vi "Autonomous Independent.vi"() -> ()   [LabVIEW 2020]
doc: "This VI is called when autonomous begins, and will automatically be terminated when autonomous ends. You can carry out timed or sensor driven robot movement independently without needing to return to the caller."
uses:
  <vilib>/Rock Robotics/WPI/ThirdParty/Phoenix-LabVIEW/Motor Controller/Controls/CTRE_Phoenix_MotorControl_ControlMode.ctl
  <vilib>/Rock Robotics/WPI/Utilities/WPI_GetSetVariantRefNum.vi
  <vilib>/Rock Robotics/Network Tables/NT Read String.vi
  <vilib>/Rock Robotics/Network Tables/NT Write Numeric Array.vi
  <vilib>/Rock Robotics/WPI/ThirdParty/Phoenix-LabVIEW/Motor Controller/Get/CTRE_Phoenix_MotorController_GetSelectedSensorData.vi
  <vilib>/Rock Robotics/WPI/RobotDrive/WPI_RobotDriveArcadeDrive_Standard(NoSaturation).vi
panel:
  out "Talon FX LEFT Moter Encoders":i32
  out "Current Movement, for debugging":T1 {"Y Joystick Value" scale=1.0..-1.0; "X Joystick Value" scale=-1.0..1.0}
  in  "Array of robot movements":T2(array[cluster])=[{"X Joystick Value"=0.39393939393939403, "Y Joystick Value"=0.0, "Delay (sec)"=1.0, "Movement Name"="turn"}, {"X Joystick Value"=-0.3737373737373737, "Y Joystick Value"=0.0, "Delay (sec)"=1.0, "Movement Name"="turn back"}] {"Y Joystick Value" scale=1.0..-1.0; "X Joystick Value" scale=-1.0..1.0}
  # "Be sure to right-click and choose Data Operations>>Make Current Value default if you want to save the array values with the VI"
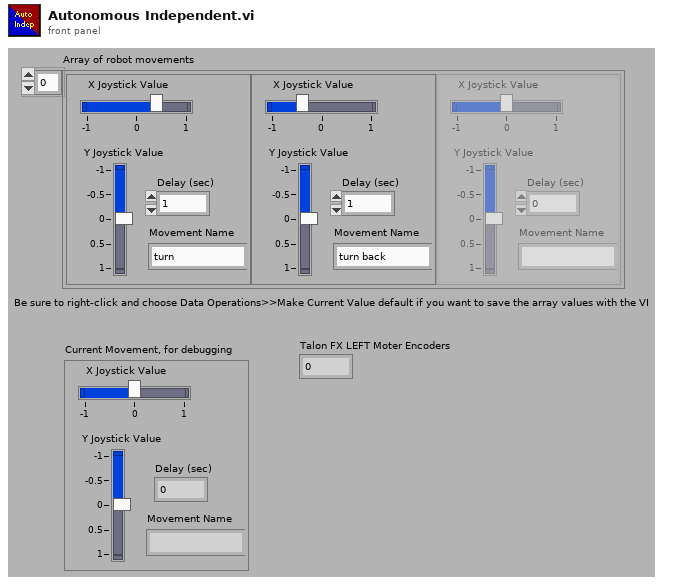
[diagram p1: front panel]
types:
  T1 = cluster{"X Joystick Value":dbl, "Y Joystick Value":dbl, "Delay (sec)":dbl, "Movement Name":string}
  T2 = cluster{"X Joystick Value":dbl, "Y Joystick Value":dbl, "Delay (sec)":dbl, "Movement Name":string}[]
  T3 = typedef "WPI_JoystickDevRef.ctl" = cluster{"Device":T4}
  T4 = typedef "WPI_JoystickDeviceEnum.ctl" = enum16{"USB 0", "USB 1", "USB 2", "USB 3", "USB 4", "USB 5"}
  T5 = typedef "WPI_MotorControlDeviceRef.ctl" = cluster{"DeviceStatus":errorcluster, "Type":T6, "PWM":cluster{"PWM Channel":T7, "DeadBand":T8}, "CAN":cluster{"Device Number":u8, "SetOutput VI Ref":variant, "GetOutput VI Ref":variant, "Enable VI Ref":variant, "Disable VI Ref":variant, "Data":variant}, "Invert":bool, "DIO PWM":cluster{"PWM \"Enable\" Channel":T7, "DIOChannel":T9, "PWM Rate":dbl}}
  T6 = typedef "WPI_MotorControlType.ctl" = enum16{"PWM", "CAN", "DIO PWM"}
  T7 = typedef "FPGA_DIOPWMChannel.ctl" = enum8{"PWM 0", "PWM 1", "PWM 2", "PWM 3", "PWM 4", "PWM 5", "PWM 6", "PWM 7", "PWM 8", "PWM 9", "PWM MXP 0", "PWM MXP 1", "PWM MXP 2", "PWM MXP 3", "PWM MXP 4", "PWM MXP 5", "PWM MXP 6", "PWM MXP 7", "PWM MXP 8", "PWM MXP 9", "Invalid"}
  T8 = typedef "WPI_PWMDeadband.ctl" = cluster{"Name":string, "maxPositivePwm":i32, "minPositivePwm":i32, "centerPwm":i32, "maxNegativePwm":i32, "minNegativePwm":i32, "angularRange":u16}
  T9 = typedef "FPGA_DIOChannel.ctl" = enum8{"DIO 0", "DIO 1", "DIO 2", "DIO 3", "DIO 4", "DIO 5", "DIO 6", "DIO 7", "DIO 8", "DIO 9", "DIO MXP 0", "DIO MXP 1", "DIO MXP 2", "DIO MXP 3", "DIO MXP 4", "DIO MXP 5", "DIO MXP 6", "DIO MXP 7", "DIO MXP 8", "DIO MXP 9", "DIO MXP 10", "DIO MXP 11", "DIO MXP 12", "DIO MXP 13", "DIO MXP 14", "DIO MXP 15", "SPI Port CS1", "SPI Port CS2", "SPI Port CS3", "SPI Port MISO", "SPI Port MOSI", "Invalid"}
  T10 = typedef "WPI_RobotDriveDevRef.ctl" = cluster{"DevStatus":errorcluster, "Motors[]":T5[], "Square Inputs":bool, "Max Output":dbl}
  T11 = typedef "CTRE_Phoenix_MotorControl_ControlMode.ctl" = u16
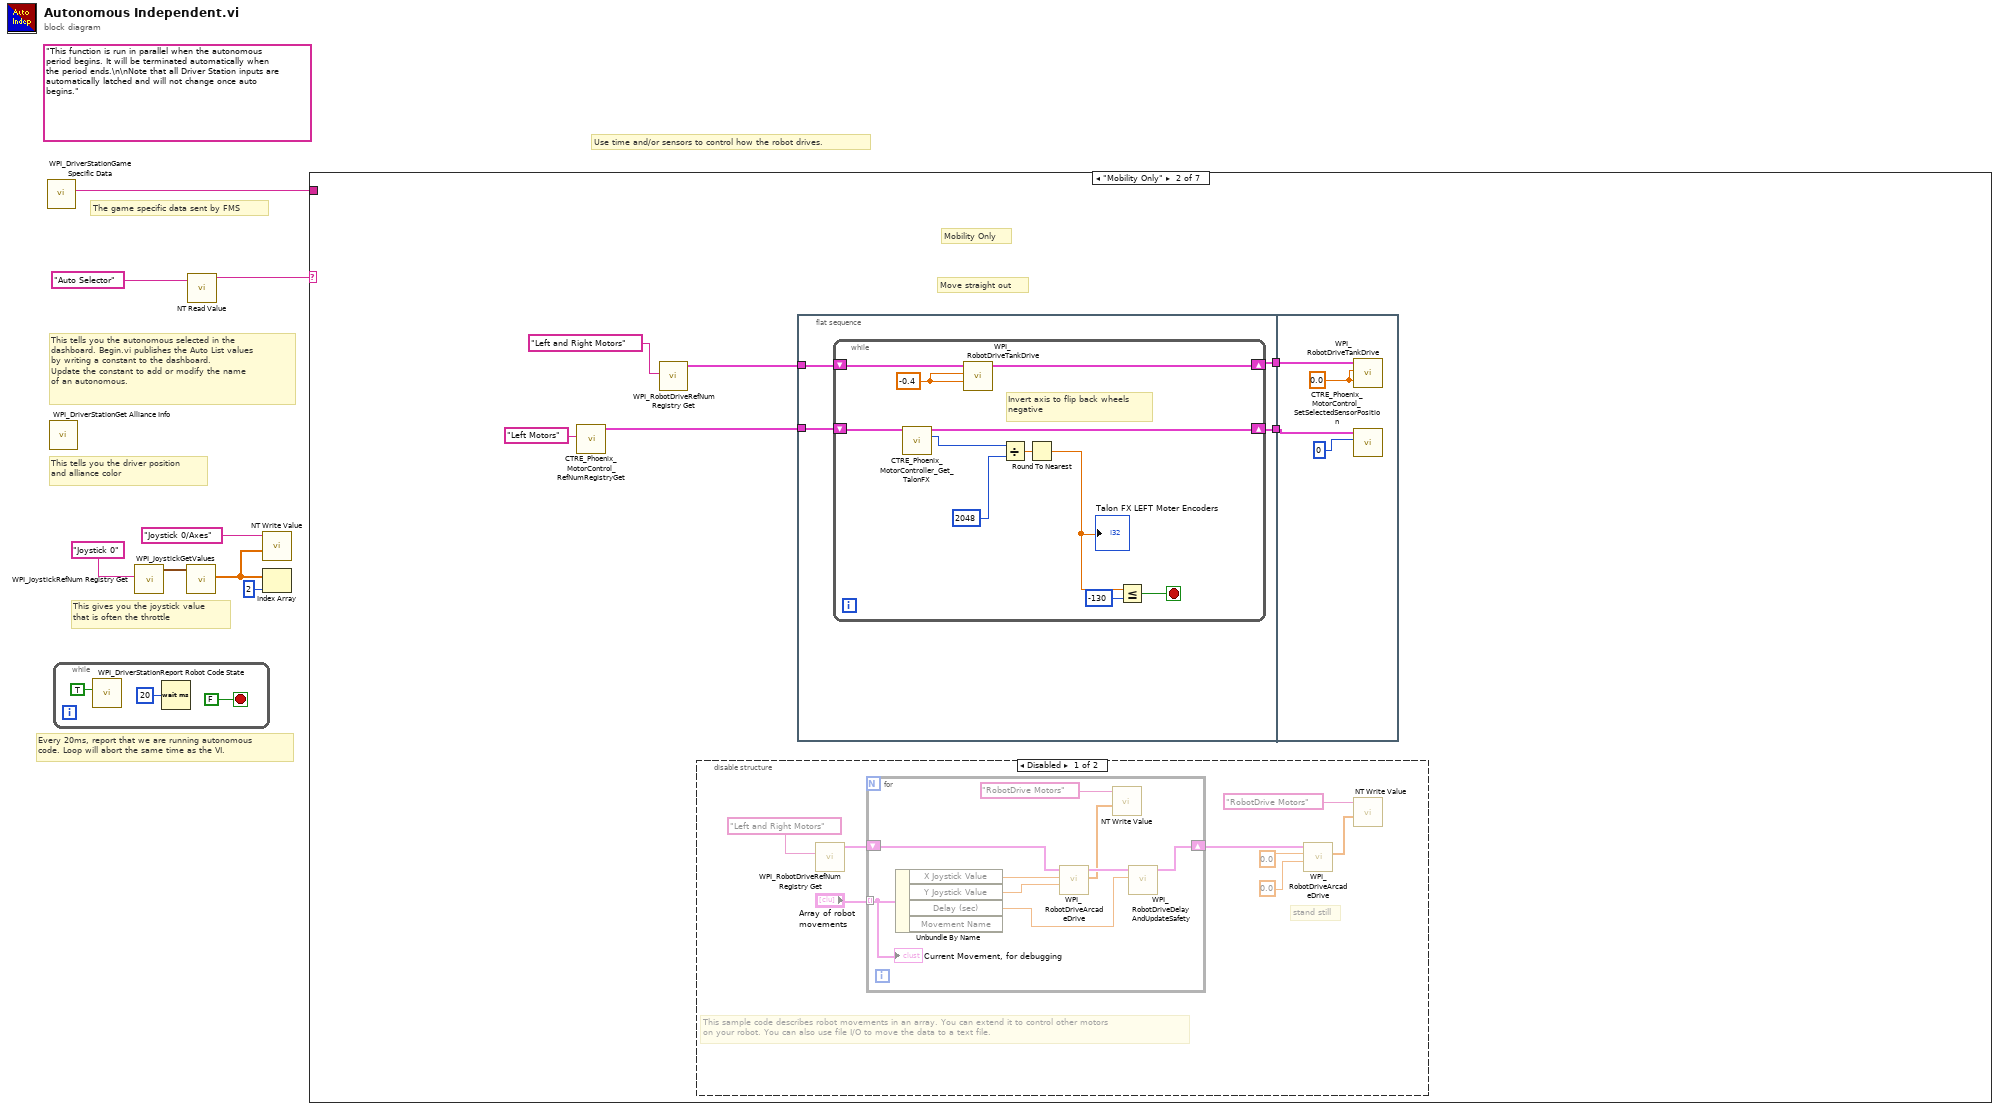
[diagram p0: block diagram]
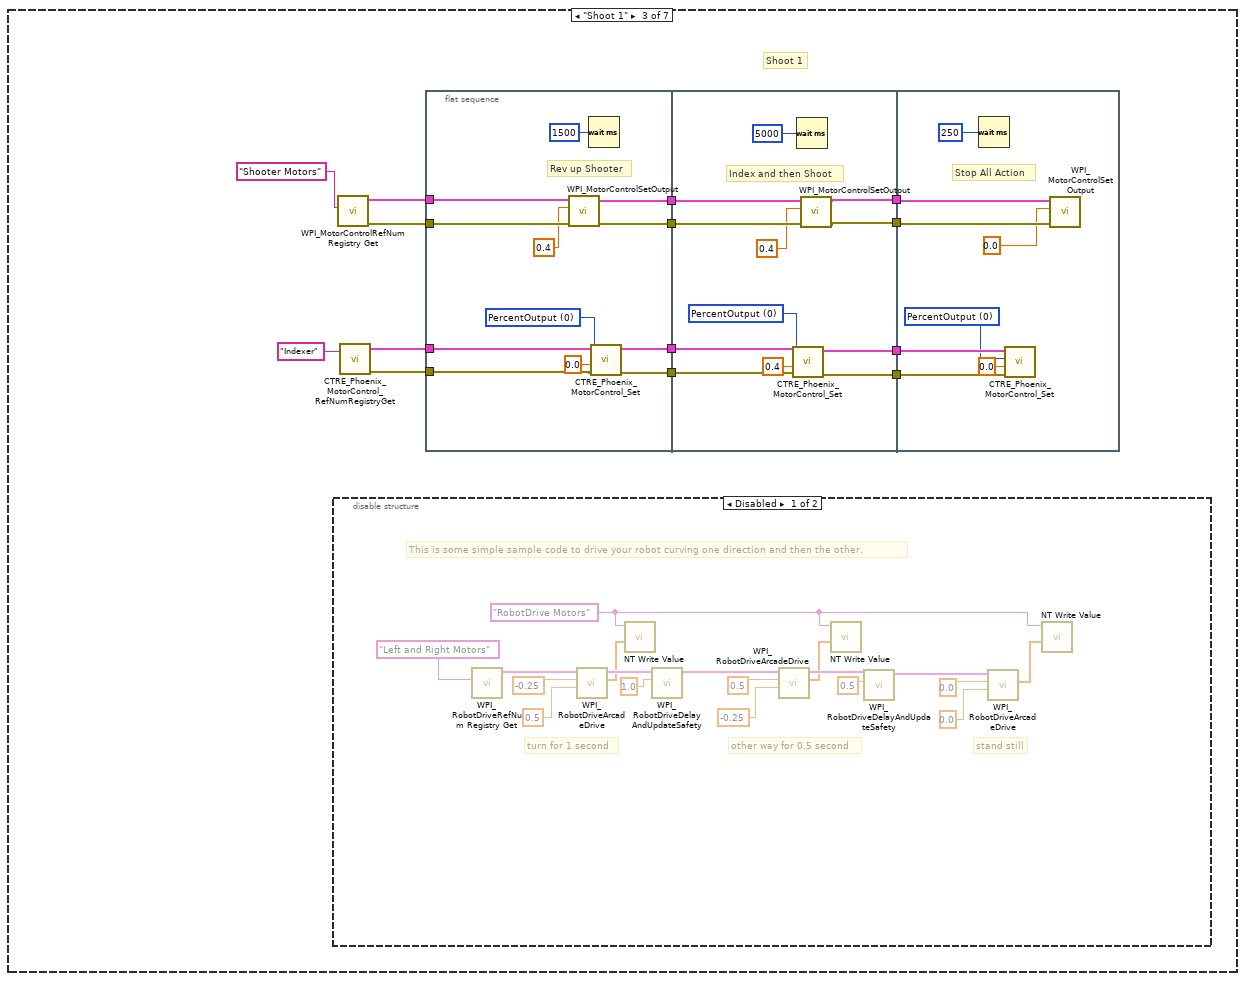
[diagram p4: hidden frame]
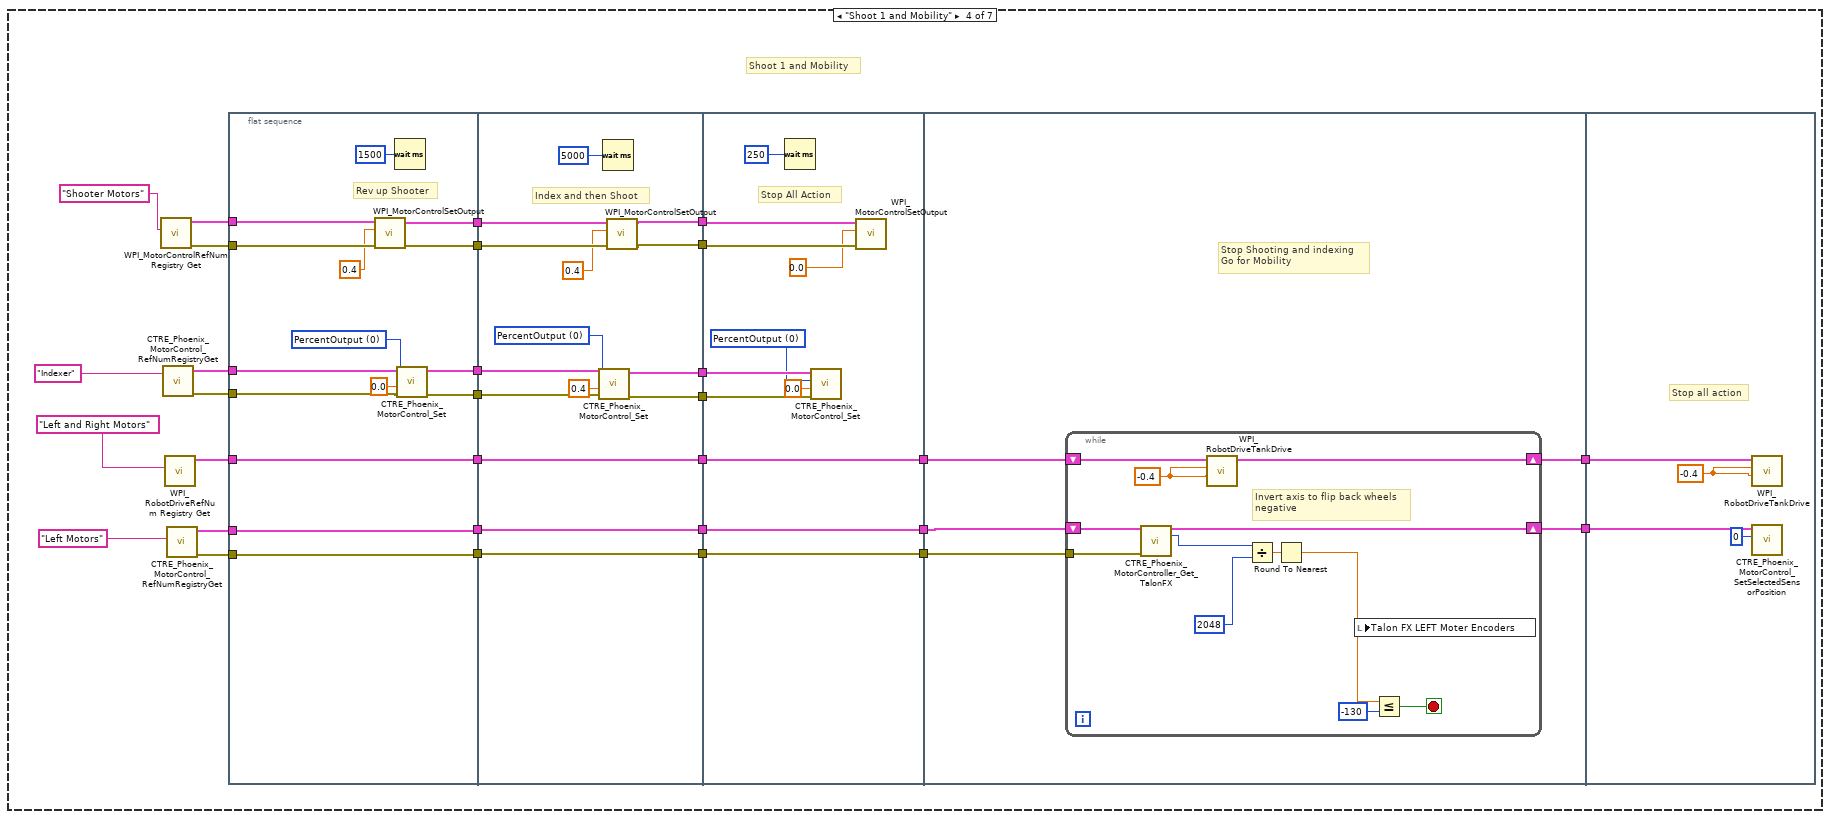
[diagram p6: hidden frame]
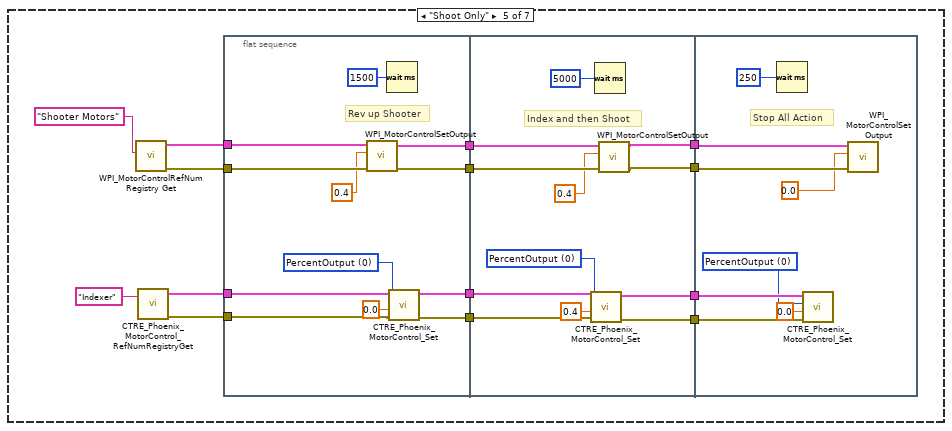
[diagram p7: hidden frame]
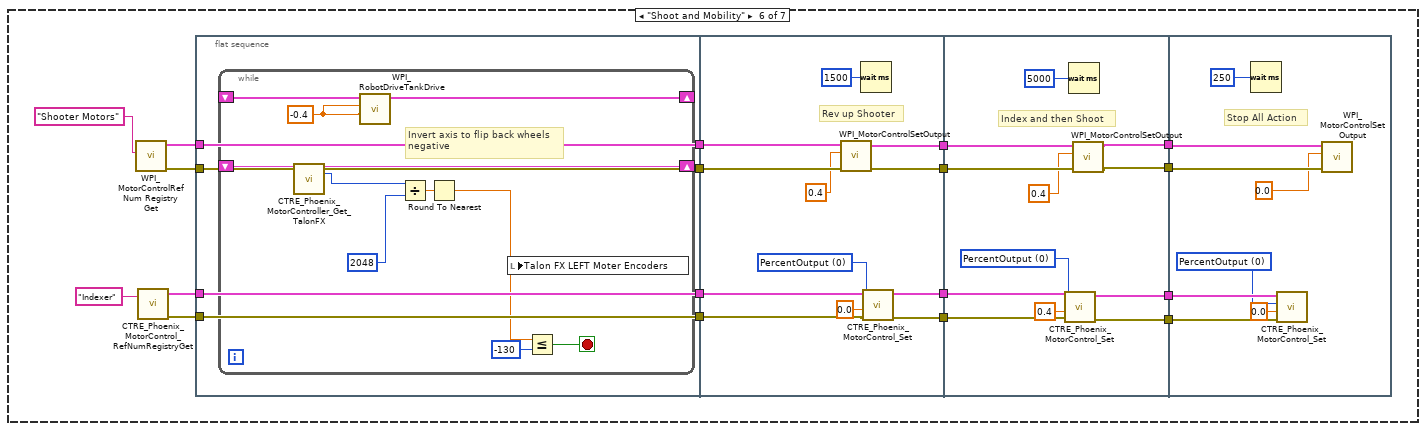
[diagram p8: hidden frame]
diagram:
  (unwired) "This function is run in parallel when the autonomous period begins. It will be terminated automatically when the period ends.\n\nNote that all Driver Station inputs are automatically latched and will not change once auto begins."
  # "The game specific data sent by FMS"
  # "This tells you the autonomous selected in the \ndashboard. Begin.vi publishes the Auto List values\nby writing a constant to the dashboard.\nUpdate the constant to add or modify the name\nof an autonomous."
  # "Every 20ms, report that we are running autonomous\ncode. Loop will abort the same time as the VI."
  # "This gives you the joystick value\nthat is often the throttle"
  # "Use time and/or sensors to control how the robot drives."
  # "This tells you the driver position\nand alliance color"
  n1 = call <vilib>:"WPI_DriverStationGame Specific Data.vi"() -> ("Game Specific Data"=w1:string)  [unwired: 11 in]
  n2 = call <vilib>:"WPI_DriverStationGet Alliance Info.vi"() -> ()  [unwired: 12 out]
  n3 = while {
    stop <- FALSE stop-if-true
    n4 = call <vilib>:"WPI_DriverStationReport Robot Code State.vi"("Autonomous"=TRUE) -> ()  [unwired: 10 in, 1 out]
    n5 = Wait (ms)(milliseconds to wait=u32 20) -> ()  [unwired: 1 out]
  }
  n6 = call <vilib>:"WPI_JoystickRefNum Registry Get.vi"("refnum name"="Joystick 0") -> ("JoystickDevRef"=w7:T3)  [unwired: 1 in, 9 out]
  n7 = call <vilib>:"WPI_JoystickGetValues.vi"("JoystickDevRef"=w7) -> ("Axes"=w3:dbl[])  [unwired: 6 in, 4 out]
  n8 = call-poly <vilib>:"NT Read Value.vi"("name"="Auto Selector" ("Name")) -> ("value"=w4:string)  [unwired: 8 in, 2 out]
  n9 = call-poly <vilib>:"NT Write Value.vi"("value"=w3, "name"="Joystick 0/Axes" ("Name")) -> ()  [unwired: 9 in, 1 out]
  n10 = Index Array(array=w3, index=2) -> ()  [unwired: 1 out]
  n11 = case shown="\"Mobility Only\"" w4 {
    tunnel: w1 -> [_ _ _ _ _ _ _]
    frame Default {
      # "You can put your main auto here, or you can right-click on the case and make any\nother frame be the default case."
      # "This is the frame that will execute if no selection is made, or if it is not recognized"
    }
    frame "Mobility Only" {
      # "Mobility Only"
      # "Move straight out"
      n12 = call <vilib>:"CTRE_Phoenix_MotorControl_RefNumRegistryGet.vi"("refnum name"="Left Motors") -> ("PhoenixMotorControlDevRef"=w14:T5)  [unwired: 9 in, 1 out]
      n13 = call <vilib>:"WPI_RobotDriveRefNum Registry Get.vi"("refnum name"="Left and Right Motors") -> ("RobotDriveDevRef"=w15:T10)  [unwired: 9 in, 1 out]
      n14 = disable-structure shown="Disabled" {
        frame Disabled {
          # "stand still"
          # "This sample code describes robot movements in an array. You can extend it to control other motors\non your robot. You can also use file I/O to move the data to a text file."
          n15 = call <vilib>:"WPI_RobotDriveRefNum Registry Get.vi"("refnum name"="Left and Right Motors") -> ("RobotDriveDevRef"=w43:T10)  [unwired: 1 in, 9 out]
          n16 = for {
            shift-right: [w51] -> w38
            shift-left: w43 -> [w52]
            tunnel: "Array of robot movements" -> [w47] mode=indexing
            n17 = Unbundle By Name(w47) -> ("X Joystick Value"=w50:dbl, "Y Joystick Value"=w49:dbl, "Delay (sec)"=w48:dbl)  [unwired: 1 out]
            n18 = call-poly <vilib>:"WPI_RobotDriveArcadeDrive.vi"("Y axis value"=w49, "X axis value"=w50, "RobotDriveDevRef"=w52) -> ("Motor Values"=w45:dbl[], "RobotDriveDevRef"=w53:T10)  [unwired: 1 in, 6 out]
            n19 = call-poly <vilib>:"NT Write Value.vi"("value"=w45, "name"="RobotDrive Motors" ("Name")) -> ()  [unwired: 9 in, 1 out]
            n20 = call <vilib>:"WPI_RobotDriveDelayAndUpdateSafety.vi"("Delay (s)"=w48, "RobotDriveDevRef"=w53) -> ("RobotDriveDevRef 2"=w51:T10)  [unwired: 8 in, 1 out]
            "Current Movement, for debugging" <- w47
          }
          n21 = call-poly <vilib>:"WPI_RobotDriveArcadeDrive.vi"("Y axis value"=0.0 ("X axis value"), "X axis value"=0.0, "RobotDriveDevRef"=w38) -> ("Motor Values"=w41:dbl[])  [unwired: 1 in, 7 out]
          n22 = call-poly <vilib>:"NT Write Value.vi"("value"=w41, "name"="RobotDrive Motors" ("Name")) -> ()  [unwired: 9 in, 1 out]
        }
        frame Enabled {
        }
      }
      n23 = flat-sequence {
        tunnel: w15 -> [w21]
        tunnel: [w20] -> w17
        tunnel: [w19] -> w16
        tunnel: w14 -> [w18]
        tunnel: w17 -> [w35]
        tunnel: w16 -> [w34]
        frame #0 {
          n24 = while {
            shift-right: [w30] -> w20
            shift-left: w21 -> [w32]
            shift-right: [w29] -> w19
            shift-left: w18 -> [w31]
            stop <- w28 stop-if-true
            w27 = -0.4 ("Left axis value")
            # "Invert axis to flip back wheels\nnegative"
            n25 = call-poly <vilib>:"CTRE_Phoenix_MotorController_Get_TalonFX.vi"("PhoenixMotorControlDevRef"=w31) -> ("PhoenixMotorControlDevRef"=w29:T5, "Position (Raw Sensor Units)"=w23:i32)  [unwired: 11 in, 2 out]
            n26 = call <vilib>:"WPI_RobotDriveTankDrive.vi"("Right axis value"=w27, "Left axis value"=w27, "RobotDriveDevRef"=w32) -> ("RobotDriveDevRef"=w30:T10)  [unwired: 6 in, 2 out]
            n27 = Divide(x=w23, y=2048) -> (x/y=w24:dbl)
            n28 = Round To Nearest(number=w24) -> (nearest integer value=w22:dbl)
            "Talon FX LEFT Moter Encoders" <- w22
            n29 = Less Or Equal?(x=w22, y=-130) -> (x <= y?=w28:bool)
          }
        }
        frame #1 {
          w36 = 0.0
          n30 = call <vilib>:"WPI_RobotDriveTankDrive.vi"("Right axis value"=w36, "Left axis value"=w36, "RobotDriveDevRef"=w35) -> ()  [unwired: 6 in, 3 out]
          n31 = call <vilib>:"CTRE_Phoenix_MotorControl_SetSelectedSensorPosition.vi"("New Sensor Position"=0, "PhoenixMotorControlDevRef"=w34) -> ()  [unwired: 8 in, 2 out]
        }
      }
    }
    frame "Shoot 1" {
      # "Shoot 1"
      n32 = disable-structure shown="Disabled" {
        frame Disabled {
          w101 = "RobotDrive Motors" ("Name")
          # "This is some simple sample code to drive your robot curving one direction and then the other."
          # "stand still"
          # "other way for 0.5 second"
          # "turn for 1 second"
          n33 = call <vilib>:"WPI_RobotDriveRefNum Registry Get.vi"("refnum name"="Left and Right Motors") -> ("RobotDriveDevRef"=w117:T10)  [unwired: 1 in, 9 out]
          n34 = call-poly <vilib>:"WPI_RobotDriveArcadeDrive.vi"("Y axis value"=0.5 ("X axis value"), "X axis value"=-0.25, "RobotDriveDevRef"=w117) -> ("Motor Values"=w100:dbl[], "RobotDriveDevRef"=w110:T10)  [unwired: 1 in, 6 out]
          n35 = call-poly <vilib>:"NT Write Value.vi"("value"=w100, "name"=w101) -> ()  [unwired: 9 in, 1 out]
          n36 = call <vilib>:"WPI_RobotDriveDelayAndUpdateSafety.vi"("Delay (s)"=1.0, "RobotDriveDevRef"=w110) -> ("RobotDriveDevRef 2"=w111:T10)  [unwired: 8 in, 1 out]
          n37 = call-poly <vilib>:"WPI_RobotDriveArcadeDrive.vi"("Y axis value"=-0.25 ("X axis value"), "X axis value"=0.5, "RobotDriveDevRef"=w111) -> ("Motor Values"=w102:dbl[], "RobotDriveDevRef"=w112:T10)  [unwired: 1 in, 6 out]
          n38 = call-poly <vilib>:"NT Write Value.vi"("value"=w102, "name"=w101) -> ()  [unwired: 9 in, 1 out]
          n39 = call <vilib>:"WPI_RobotDriveDelayAndUpdateSafety.vi"("Delay (s)"=0.5, "RobotDriveDevRef"=w112) -> ("RobotDriveDevRef 2"=w113:T10)  [unwired: 8 in, 1 out]
          n40 = call-poly <vilib>:"WPI_RobotDriveArcadeDrive.vi"("Y axis value"=0.0 ("X axis value"), "X axis value"=0.0, "RobotDriveDevRef"=w113) -> ("Motor Values"=w103:dbl[])  [unwired: 1 in, 7 out]
          n41 = call-poly <vilib>:"NT Write Value.vi"("value"=w103, "name"=w101) -> ()  [unwired: 9 in, 1 out]
        }
        frame Enabled {
        }
      }
      n42 = call <vilib>:"WPI_MotorControlRefNum Registry Get.vi"("refnum name"="Shooter Motors") -> ("error out"=w56:errorcluster, "MotorControlDevRef"=w57:T5)  [unwired: 9 in]
      n43 = call <vilib>:"CTRE_Phoenix_MotorControl_RefNumRegistryGet.vi"("refnum name"="Indexer") -> ("error out"=w58:errorcluster, "PhoenixMotorControlDevRef"=w59:T5)  [unwired: 9 in]
      n44 = flat-sequence {
        tunnel: w57 -> [w79]
        tunnel: w56 -> [w78]
        tunnel: [w75] -> w67
        tunnel: [w74] -> w66
        tunnel: [w73] -> w65
        tunnel: [w72] -> w64
        tunnel: w59 -> [w71]
        tunnel: w58 -> [w70]
        tunnel: w67 -> [w90]
        tunnel: w66 -> [w89]
        tunnel: [w88] -> w63
        tunnel: [w87] -> w62
        tunnel: [w85] -> w61
        tunnel: [w84] -> w60
        tunnel: w65 -> [w83]
        tunnel: w64 -> [w82]
        tunnel: w63 -> [w99]
        tunnel: w62 -> [w98]
        tunnel: w61 -> [w95]
        tunnel: w60 -> [w94]
        frame #0 {
          w68 = T11 0 items=["PercentOutput"=0, "Position"=1, "Velocity"=2, "Current"=3, "Follower"=5, "MotionProfile"=6, "MotionMagic"=7, "MotionProfileArc"=10, "Disabled"=15] ("Control Mode")
          # "Rev up Shooter"
          n45 = call <vilib>:"WPI_MotorControlSetOutput.vi"("error in (no error)"=w78, "Output"=0.4, "MotorControlDevRef"=w79) -> ("error out"=w74:errorcluster, "MotorControlDevRef"=w75:T5)  [unwired: 6 in, 1 out]
          n46 = Wait (ms)(milliseconds to wait=u32 1500) -> ()  [unwired: 1 out]
          n47 = call <vilib>:"CTRE_Phoenix_MotorControl_Set.vi"("error in (no error)"=w70, "Output"=0.0, "Control Mode"=w68, "PhoenixMotorControlDevRef"=w71) -> ("error out"=w72:errorcluster, "PhoenixMotorControlDevRef"=w73:T5)  [unwired: 6 in]
        }
        frame #1 {
          w80 = T11 0 items=["PercentOutput"=0, "Position"=1, "Velocity"=2, "Current"=3, "Follower"=5, "MotionProfile"=6, "MotionMagic"=7, "MotionProfileArc"=10, "Disabled"=15] ("Control Mode")
          # "Index and then Shoot"
          n48 = call <vilib>:"CTRE_Phoenix_MotorControl_Set.vi"("error in (no error)"=w82, "Output"=0.4, "Control Mode"=w80, "PhoenixMotorControlDevRef"=w83) -> ("error out"=w84:errorcluster, "PhoenixMotorControlDevRef"=w85:T5)  [unwired: 6 in]
          n49 = Wait (ms)(milliseconds to wait=u32 5000) -> ()  [unwired: 1 out]
          n50 = call <vilib>:"WPI_MotorControlSetOutput.vi"("error in (no error)"=w89, "Output"=0.4, "MotorControlDevRef"=w90) -> ("error out"=w87:errorcluster, "MotorControlDevRef"=w88:T5)  [unwired: 6 in, 1 out]
        }
        frame #2 {
          w92 = T11 0 items=["PercentOutput"=0, "Position"=1, "Velocity"=2, "Current"=3, "Follower"=5, "MotionProfile"=6, "MotionMagic"=7, "MotionProfileArc"=10, "Disabled"=15] ("Control Mode")
          # "Stop All Action"
          n51 = Wait (ms)(milliseconds to wait=u32 250) -> ()  [unwired: 1 out]
          n52 = call <vilib>:"CTRE_Phoenix_MotorControl_Set.vi"("error in (no error)"=w94, "Output"=0.0, "Control Mode"=w92, "PhoenixMotorControlDevRef"=w95) -> ()  [unwired: 6 in, 2 out]
          n53 = call <vilib>:"WPI_MotorControlSetOutput.vi"("error in (no error)"=w98, "Output"=0.0, "MotorControlDevRef"=w99) -> ()  [unwired: 6 in, 3 out]
        }
      }
    }
    frame "Shoot 1 and Mobility" {
      # "Shoot 1 and Mobility"
      n54 = call <vilib>:"WPI_MotorControlRefNum Registry Get.vi"("refnum name"="Shooter Motors") -> ("error out"=w136:errorcluster, "MotorControlDevRef"=w137:T5)  [unwired: 9 in]
      n55 = call <vilib>:"CTRE_Phoenix_MotorControl_RefNumRegistryGet.vi"("refnum name"="Indexer") -> ("error out"=w138:errorcluster, "PhoenixMotorControlDevRef"=w139:T5)  [unwired: 9 in]
      n56 = call <vilib>:"WPI_RobotDriveRefNum Registry Get.vi"("refnum name"="Left and Right Motors") -> ("RobotDriveDevRef"=w130:T10)  [unwired: 9 in, 1 out]
      n57 = call <vilib>:"CTRE_Phoenix_MotorControl_RefNumRegistryGet.vi"("refnum name"="Left Motors") -> ("error out"=w122:errorcluster, "PhoenixMotorControlDevRef"=w126:T5)  [unwired: 9 in]
      n58 = flat-sequence {
        tunnel: [w158] -> w147
        tunnel: [w157] -> w146
        tunnel: [w156] -> w145
        tunnel: [w155] -> w144
        tunnel: w137 -> [w162]
        tunnel: w136 -> [w161]
        tunnel: w139 -> [w154]
        tunnel: w138 -> [w153]
        tunnel: [w150] -> w131
        tunnel: w130 -> [w150]
        tunnel: [w149] -> w127
        tunnel: w126 -> [w149]
        tunnel: [w148] -> w123
        tunnel: w122 -> [w148]
        tunnel: w147 -> [w176]
        tunnel: w146 -> [w175]
        tunnel: [w174] -> w143
        tunnel: [w173] -> w142
        tunnel: [w171] -> w141
        tunnel: [w170] -> w140
        tunnel: w145 -> [w169]
        tunnel: w144 -> [w168]
        tunnel: w131 -> [w165]
        tunnel: [w165] -> w129
        tunnel: w127 -> [w164]
        tunnel: [w164] -> w125
        tunnel: w123 -> [w163]
        tunnel: [w163] -> w120
        tunnel: w143 -> [w188]
        tunnel: w142 -> [w187]
        tunnel: w141 -> [w184]
        tunnel: w140 -> [w183]
        tunnel: w129 -> [w180]
        tunnel: [w180] -> w128
        tunnel: w125 -> [w179]
        tunnel: [w179] -> w124
        tunnel: [w178] -> w121
        tunnel: w120 -> [w178]
        tunnel: w128 -> [w193]
        tunnel: w124 -> [w192]
        tunnel: w121 -> [w191]
        tunnel: [w190] -> w119
        tunnel: [w189] -> w118
        tunnel: w119 -> [w208]
        tunnel: w118 -> [w207]
        frame #0 {
          w151 = T11 0 items=["PercentOutput"=0, "Position"=1, "Velocity"=2, "Current"=3, "Follower"=5, "MotionProfile"=6, "MotionMagic"=7, "MotionProfileArc"=10, "Disabled"=15] ("Control Mode")
          # "Rev up Shooter"
          n59 = call <vilib>:"WPI_MotorControlSetOutput.vi"("error in (no error)"=w161, "Output"=0.4, "MotorControlDevRef"=w162) -> ("error out"=w157:errorcluster, "MotorControlDevRef"=w158:T5)  [unwired: 6 in, 1 out]
          n60 = Wait (ms)(milliseconds to wait=u32 1500) -> ()  [unwired: 1 out]
          n61 = call <vilib>:"CTRE_Phoenix_MotorControl_Set.vi"("error in (no error)"=w153, "Output"=0.0, "Control Mode"=w151, "PhoenixMotorControlDevRef"=w154) -> ("error out"=w155:errorcluster, "PhoenixMotorControlDevRef"=w156:T5)  [unwired: 6 in]
        }
        frame #1 {
          w166 = T11 0 items=["PercentOutput"=0, "Position"=1, "Velocity"=2, "Current"=3, "Follower"=5, "MotionProfile"=6, "MotionMagic"=7, "MotionProfileArc"=10, "Disabled"=15] ("Control Mode")
          # "Index and then Shoot"
          n62 = call <vilib>:"CTRE_Phoenix_MotorControl_Set.vi"("error in (no error)"=w168, "Output"=0.4, "Control Mode"=w166, "PhoenixMotorControlDevRef"=w169) -> ("error out"=w170:errorcluster, "PhoenixMotorControlDevRef"=w171:T5)  [unwired: 6 in]
          n63 = Wait (ms)(milliseconds to wait=u32 5000) -> ()  [unwired: 1 out]
          n64 = call <vilib>:"WPI_MotorControlSetOutput.vi"("error in (no error)"=w175, "Output"=0.4, "MotorControlDevRef"=w176) -> ("error out"=w173:errorcluster, "MotorControlDevRef"=w174:T5)  [unwired: 6 in, 1 out]
        }
        frame #2 {
          w181 = T11 0 items=["PercentOutput"=0, "Position"=1, "Velocity"=2, "Current"=3, "Follower"=5, "MotionProfile"=6, "MotionMagic"=7, "MotionProfileArc"=10, "Disabled"=15] ("Control Mode")
          # "Stop All Action"
          n65 = Wait (ms)(milliseconds to wait=u32 250) -> ()  [unwired: 1 out]
          n66 = call <vilib>:"CTRE_Phoenix_MotorControl_Set.vi"("error in (no error)"=w183, "Output"=0.0, "Control Mode"=w181, "PhoenixMotorControlDevRef"=w184) -> ()  [unwired: 6 in, 2 out]
          n67 = call <vilib>:"WPI_MotorControlSetOutput.vi"("error in (no error)"=w187, "Output"=0.0, "MotorControlDevRef"=w188) -> ()  [unwired: 6 in, 3 out]
        }
        frame #3 {
          # "Stop Shooting and indexing\nGo for Mobility"
          n68 = while {
            shift-right: [w203] -> w190
            shift-left: w193 -> [w205]
            shift-right: [w202] -> w189
            shift-left: w192 -> [w204]
            tunnel: w191 -> [w194]
            stop <- w201 stop-if-true
            w200 = -0.4 ("Left axis value")
            # "Invert axis to flip back wheels\nnegative"
            n69 = call-poly <vilib>:"CTRE_Phoenix_MotorController_Get_TalonFX.vi"("PhoenixMotorControlDevRef"=w204, "error in"=w194) -> ("PhoenixMotorControlDevRef"=w202:T5, "Position (Raw Sensor Units)"=w196:i32)  [unwired: 10 in, 2 out]
            n70 = call <vilib>:"WPI_RobotDriveTankDrive.vi"("Right axis value"=w200, "Left axis value"=w200, "RobotDriveDevRef"=w205) -> ("RobotDriveDevRef"=w203:T10)  [unwired: 6 in, 2 out]
            n71 = Divide(x=w196, y=2048) -> (x/y=w197:dbl)
            n72 = Round To Nearest(number=w197) -> (nearest integer value=w195:dbl)
            n73 = local write "Talon FX LEFT Moter Encoders"(w195) -> ()
            n74 = Less Or Equal?(x=w195, y=-130) -> (x <= y?=w201:bool)
          }
        }
        frame #4 {
          w209 = -0.4 ("Left axis value")
          # "Stop all action"
          n75 = call <vilib>:"WPI_RobotDriveTankDrive.vi"("Right axis value"=w209, "Left axis value"=w209, "RobotDriveDevRef"=w208) -> ()  [unwired: 6 in, 3 out]
          n76 = call <vilib>:"CTRE_Phoenix_MotorControl_SetSelectedSensorPosition.vi"("New Sensor Position"=0, "PhoenixMotorControlDevRef"=w207) -> ()  [unwired: 8 in, 2 out]
        }
      }
    }
    frame "Shoot Only" {
      n77 = call <vilib>:"WPI_MotorControlRefNum Registry Get.vi"("refnum name"="Shooter Motors") -> ("error out"=w212:errorcluster, "MotorControlDevRef"=w213:T5)  [unwired: 9 in]
      n78 = call <vilib>:"CTRE_Phoenix_MotorControl_RefNumRegistryGet.vi"("refnum name"="Indexer") -> ("error out"=w214:errorcluster, "PhoenixMotorControlDevRef"=w215:T5)  [unwired: 9 in]
      n79 = flat-sequence {
        tunnel: w213 -> [w235]
        tunnel: w212 -> [w234]
        tunnel: [w231] -> w223
        tunnel: [w230] -> w222
        tunnel: [w229] -> w217
        tunnel: [w228] -> w216
        tunnel: w215 -> [w227]
        tunnel: w214 -> [w226]
        tunnel: w223 -> [w246]
        tunnel: w222 -> [w245]
        tunnel: [w244] -> w221
        tunnel: [w243] -> w220
        tunnel: [w241] -> w219
        tunnel: [w240] -> w218
        tunnel: w217 -> [w239]
        tunnel: w216 -> [w238]
        tunnel: w221 -> [w255]
        tunnel: w220 -> [w254]
        tunnel: w219 -> [w251]
        tunnel: w218 -> [w250]
        frame #0 {
          w224 = T11 0 items=["PercentOutput"=0, "Position"=1, "Velocity"=2, "Current"=3, "Follower"=5, "MotionProfile"=6, "MotionMagic"=7, "MotionProfileArc"=10, "Disabled"=15] ("Control Mode")
          # "Rev up Shooter"
          n80 = call <vilib>:"WPI_MotorControlSetOutput.vi"("error in (no error)"=w234, "Output"=0.4, "MotorControlDevRef"=w235) -> ("error out"=w230:errorcluster, "MotorControlDevRef"=w231:T5)  [unwired: 6 in, 1 out]
          n81 = Wait (ms)(milliseconds to wait=u32 1500) -> ()  [unwired: 1 out]
          n82 = call <vilib>:"CTRE_Phoenix_MotorControl_Set.vi"("error in (no error)"=w226, "Output"=0.0, "Control Mode"=w224, "PhoenixMotorControlDevRef"=w227) -> ("error out"=w228:errorcluster, "PhoenixMotorControlDevRef"=w229:T5)  [unwired: 6 in]
        }
        frame #1 {
          w236 = T11 0 items=["PercentOutput"=0, "Position"=1, "Velocity"=2, "Current"=3, "Follower"=5, "MotionProfile"=6, "MotionMagic"=7, "MotionProfileArc"=10, "Disabled"=15] ("Control Mode")
          # "Index and then Shoot"
          n83 = call <vilib>:"CTRE_Phoenix_MotorControl_Set.vi"("error in (no error)"=w238, "Output"=0.4, "Control Mode"=w236, "PhoenixMotorControlDevRef"=w239) -> ("error out"=w240:errorcluster, "PhoenixMotorControlDevRef"=w241:T5)  [unwired: 6 in]
          n84 = Wait (ms)(milliseconds to wait=u32 5000) -> ()  [unwired: 1 out]
          n85 = call <vilib>:"WPI_MotorControlSetOutput.vi"("error in (no error)"=w245, "Output"=0.4, "MotorControlDevRef"=w246) -> ("error out"=w243:errorcluster, "MotorControlDevRef"=w244:T5)  [unwired: 6 in, 1 out]
        }
        frame #2 {
          w248 = T11 0 items=["PercentOutput"=0, "Position"=1, "Velocity"=2, "Current"=3, "Follower"=5, "MotionProfile"=6, "MotionMagic"=7, "MotionProfileArc"=10, "Disabled"=15] ("Control Mode")
          # "Stop All Action"
          n86 = Wait (ms)(milliseconds to wait=u32 250) -> ()  [unwired: 1 out]
          n87 = call <vilib>:"CTRE_Phoenix_MotorControl_Set.vi"("error in (no error)"=w250, "Output"=0.0, "Control Mode"=w248, "PhoenixMotorControlDevRef"=w251) -> ()  [unwired: 6 in, 2 out]
          n88 = call <vilib>:"WPI_MotorControlSetOutput.vi"("error in (no error)"=w254, "Output"=0.0, "MotorControlDevRef"=w255) -> ()  [unwired: 6 in, 3 out]
        }
      }
    }
    frame "Shoot and Mobility" {
      n89 = call <vilib>:"WPI_MotorControlRefNum Registry Get.vi"("refnum name"="Shooter Motors") -> ("error out"=w262:errorcluster, "MotorControlDevRef"=w263:T5)  [unwired: 9 in]
      n90 = call <vilib>:"CTRE_Phoenix_MotorControl_RefNumRegistryGet.vi"("refnum name"="Indexer") -> ("error out"=w264:errorcluster, "PhoenixMotorControlDevRef"=w265:T5)  [unwired: 9 in]
      n91 = flat-sequence {
        tunnel: w264 -> [w274]
        tunnel: w265 -> [w275]
        tunnel: w262 -> [w276]
        tunnel: w263 -> [w277]
        tunnel: [w277] -> w259
        tunnel: [w276] -> w258
        tunnel: [w275] -> w257
        tunnel: [w274] -> w256
        tunnel: [w296] -> w273
        tunnel: [w295] -> w272
        tunnel: [w294] -> w271
        tunnel: [w293] -> w270
        tunnel: w259 -> [w300]
        tunnel: w258 -> [w299]
        tunnel: w257 -> [w292]
        tunnel: w256 -> [w291]
        tunnel: w273 -> [w311]
        tunnel: w272 -> [w310]
        tunnel: [w309] -> w269
        tunnel: [w308] -> w268
        tunnel: [w306] -> w267
        tunnel: [w305] -> w266
        tunnel: w271 -> [w304]
        tunnel: w270 -> [w303]
        tunnel: w269 -> [w320]
        tunnel: w268 -> [w319]
        tunnel: w267 -> [w316]
        tunnel: w266 -> [w315]
        frame #0 {
          n92 = while {
            shift-right: [w286] -> _
            shift-left: _ -> [w288]
            shift-right: [w285] -> _
            shift-left: _ -> [w287]
            stop <- w284 stop-if-true
            w283 = -0.4 ("Left axis value")
            # "Invert axis to flip back wheels\nnegative"
            n93 = call-poly <vilib>:"CTRE_Phoenix_MotorController_Get_TalonFX.vi"("PhoenixMotorControlDevRef"=w287) -> ("PhoenixMotorControlDevRef"=w285:T5, "Position (Raw Sensor Units)"=w279:i32)  [unwired: 11 in, 2 out]
            n94 = call <vilib>:"WPI_RobotDriveTankDrive.vi"("Right axis value"=w283, "Left axis value"=w283, "RobotDriveDevRef"=w288) -> ("RobotDriveDevRef"=w286:T10)  [unwired: 6 in, 2 out]
            n95 = Divide(x=w279, y=2048) -> (x/y=w280:dbl)
            n96 = Round To Nearest(number=w280) -> (nearest integer value=w278:dbl)
            n97 = local write "Talon FX LEFT Moter Encoders"(w278) -> ()
            n98 = Less Or Equal?(x=w278, y=-130) -> (x <= y?=w284:bool)
          }
        }
        frame #1 {
          w289 = T11 0 items=["PercentOutput"=0, "Position"=1, "Velocity"=2, "Current"=3, "Follower"=5, "MotionProfile"=6, "MotionMagic"=7, "MotionProfileArc"=10, "Disabled"=15] ("Control Mode")
          # "Rev up Shooter"
          n99 = call <vilib>:"WPI_MotorControlSetOutput.vi"("error in (no error)"=w299, "Output"=0.4, "MotorControlDevRef"=w300) -> ("error out"=w295:errorcluster, "MotorControlDevRef"=w296:T5)  [unwired: 6 in, 1 out]
          n100 = Wait (ms)(milliseconds to wait=u32 1500) -> ()  [unwired: 1 out]
          n101 = call <vilib>:"CTRE_Phoenix_MotorControl_Set.vi"("error in (no error)"=w291, "Output"=0.0, "Control Mode"=w289, "PhoenixMotorControlDevRef"=w292) -> ("error out"=w293:errorcluster, "PhoenixMotorControlDevRef"=w294:T5)  [unwired: 6 in]
        }
        frame #2 {
          w301 = T11 0 items=["PercentOutput"=0, "Position"=1, "Velocity"=2, "Current"=3, "Follower"=5, "MotionProfile"=6, "MotionMagic"=7, "MotionProfileArc"=10, "Disabled"=15] ("Control Mode")
          # "Index and then Shoot"
          n102 = call <vilib>:"CTRE_Phoenix_MotorControl_Set.vi"("error in (no error)"=w303, "Output"=0.4, "Control Mode"=w301, "PhoenixMotorControlDevRef"=w304) -> ("error out"=w305:errorcluster, "PhoenixMotorControlDevRef"=w306:T5)  [unwired: 6 in]
          n103 = Wait (ms)(milliseconds to wait=u32 5000) -> ()  [unwired: 1 out]
          n104 = call <vilib>:"WPI_MotorControlSetOutput.vi"("error in (no error)"=w310, "Output"=0.4, "MotorControlDevRef"=w311) -> ("error out"=w308:errorcluster, "MotorControlDevRef"=w309:T5)  [unwired: 6 in, 1 out]
        }
        frame #3 {
          w313 = T11 0 items=["PercentOutput"=0, "Position"=1, "Velocity"=2, "Current"=3, "Follower"=5, "MotionProfile"=6, "MotionMagic"=7, "MotionProfileArc"=10, "Disabled"=15] ("Control Mode")
          # "Stop All Action"
          n105 = Wait (ms)(milliseconds to wait=u32 250) -> ()  [unwired: 1 out]
          n106 = call <vilib>:"CTRE_Phoenix_MotorControl_Set.vi"("error in (no error)"=w315, "Output"=0.0, "Control Mode"=w313, "PhoenixMotorControlDevRef"=w316) -> ()  [unwired: 6 in, 2 out]
          n107 = call <vilib>:"WPI_MotorControlSetOutput.vi"("error in (no error)"=w319, "Output"=0.0, "MotorControlDevRef"=w320) -> ()  [unwired: 6 in, 3 out]
        }
      }
    }
    frame "Your Turn" {
    }
  }
